vi "TrapProfile_IsFinished.vi"(9 "Time":dbl format="%20.4f", 11 "TRAPEZOID_PROFILE":T1 {"Goal"."Velocity" format="%16_6e"; "Goal"."Position" format="%16_6e"; "Initial"."Velocity" format="%16_6e"; "Initial"."Position" format="%16_6e"; "Constraints"."MaxAcceleration" format="%16_6e"; "Constraints"."MaxVelocity" format="%16_6e"; "EndDecel" format="%16_6e"; "EndFullSpeed" format="%16_6e"; "EndAccel" format="%16_6e"}) -> (3 "Finished":bool)   [LabVIEW 2019, in "Trajectory_Library.lvlib"]
doc: "Returns true if the profile has reached the goal.\n \nThe profile has reached the goal if the time since the profile started has exceeded the profile's total time.\n \nInputs:\n - Trapezoid_Profile -- The Trapezoid_Profile data cluster\n - t -- The time since the beginning of the profile.\n\nOutputs:\n - Finished -- True if the profile has reached the goal based soley on time being exceeded."
uses:
  Trajectory_Library.lvlib
  TypeDef/TRAPEZOID_PROFILE_CONSTRAINT.ctl
  TypeDef/TRAPEZOID_PROFILE_STATE.ctl
  TypeDef/TRAPEZOID_PROFILE.ctl
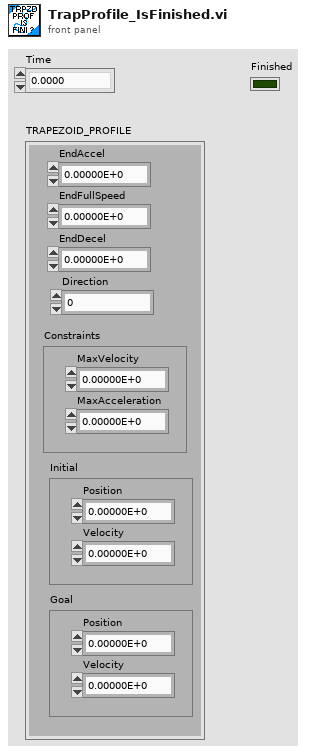
[diagram p1: front panel]
types:
  T1 = typedef "Trajectory_Library.lvlib/TRAPEZOID_PROFILE.ctl" = cluster{"EndAccel":dbl, "EndFullSpeed":dbl, "EndDecel":dbl, "Direction":i32, "Constraints":T2, "Initial":T3, "Goal":T3}
  T2 = typedef "Trajectory_Library.lvlib/TRAPEZOID_PROFILE_CONSTRAINT.ctl" = cluster{"MaxVelocity":dbl, "MaxAcceleration":dbl}
  T3 = typedef "Trajectory_Library.lvlib/TRAPEZOID_PROFILE_STATE.ctl" = cluster{"Position":dbl, "Velocity":dbl}
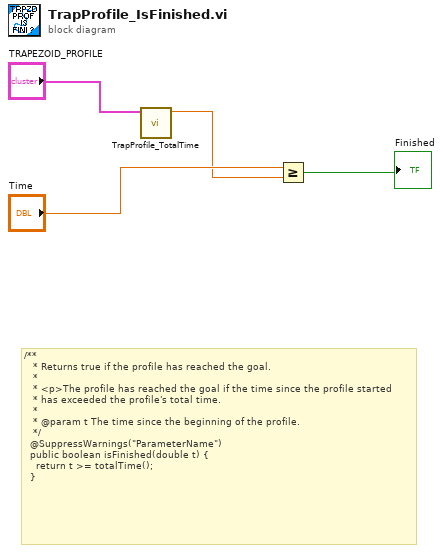
[diagram p0: block diagram]
diagram:
  # "/**\n   * Returns true if the profile has reached the goal.\n   *\n   * <p>The profile has reached the goal if the time since the profile started\n   * has exceeded the profile's total time.\n   *\n   * @param t The time since the beginning of the profile.\n   */\n  @SuppressWarnings(\"ParameterName\")\n  public boolean isFinished(double t) {\n    return t >= totalTime();\n  }"
  n1 = call "TrapProfile_TotalTime.vi"("TRAPEZOID_PROFILE"="TRAPEZOID_PROFILE") -> ("TotalTime"=w1:dbl)  [unwired: 10 in]
  n2 = Greater Or Equal?(x="Time", y=w1) -> (x >= y?=→"Finished":bool)
